vi "Digital chip test.vi"() -> ()   [LabVIEW 2019]
uses:
  <vilib>/Utility/error.llb/DialogType.ctl
  <vilib>/VirtualBench/_DMM Configure Measurement2.vi
  <vilib>/VirtualBench/_PS Configure Voltage Output0.vi
  <vilib>/VirtualBench/_FGEN Configure Standard Waveform4.vi
  <vilib>/VirtualBench/_MSO Configure Analog Channel28.vi
  <vilib>/VirtualBench/_MSO Configure Timing12.vi
  <vilib>/VirtualBench/VirtualBench.lvlib
  <vilib>/DigilentWF/DigilentWF.lvlib
panel:
  out "VOL(V)":dbl=0.31394030101314113 format="%#.2f"
  in  "图表选项卡":enum32{"VOH", "VOL", "电压传输特性"}(tab)=enum."电压传输特性"
  out "VOH":string[][](table)=[["4.750000", "0.100000", "-400.366771", "3.323930"]]
  out "VOL(V)":string[][](table)=[["4.750000", "0.100000", "1.870034", "0.313940"]]
  out "波形图":waveform(dbl)[](graph)=[{"t0"=timestamp(3807570457.144273 s since 1904-01-01), "dt"=1e-06, "Y"=array[5001 elements], "attributes"=variant("NI_ChannelName"=variant(string "mso/1"), "NI_UnitDescription"=variant(string "Volts"))}, {"t0"=timestamp(3807570457.144273 s since 1904-01-01), "dt"=1e-06, "Y"=array[5001 elements], "attributes"=variant("NI_ChannelName"=variant(string "mso/2"), "NI_UnitDescription"=variant(string "Volts"))}]
  out "VOH(V)":dbl=3.3239303310872046 format="%#.2f"
  out "IIH(μA)":dbl=1.1257554185044154 format="%#.2f"
  out "IIL(mA)":dbl=-0.1878597460447979 format="%#.2f"
  out "ICCH(mA)":dbl=0.8908473136992855 format="%#.2f"
  in  "测试参数选项卡":T1(tab)=enum."VOL"
  in  "通道一电压":T2={"+6V通道"="ADP5250-32C0AAE/ps/+6V", "Voltage Level"=5.25, "Current Limit"=0.1}
  in  "测量模式":T3(ring)=enum."DC Current"
  in  "通道一电压 2":T2={"+6V通道"="ADP5250-32C0AAE/ps/+6V", "Voltage Level"=5.25, "Current Limit"=0.1}
  in  "测量模式":T3(ring)=enum."DC Current"
  in  "通道一电压":T2={"+6V通道"="ADP5250-32C0AAE/ps/+6V", "Voltage Level"=5.25, "Current Limit"=0.1}
  in  "测量模式":T3(ring)=enum."DC Current"
  in  "通道一电压 3":T4={"+25V通道"="ADP5250-32C0AAE/ps/+25V", "Voltage Level"=0.4, "Current Limit"=0.1}
  in  "通道一电压":T2={"+6V通道"="ADP5250-32C0AAE/ps/+6V", "Voltage Level"=5.25, "Current Limit"=0.1}
  in  "测量模式":T3(ring)=enum."DC Current"
  in  "通道一电压2":T4={"+25V通道"="ADP5250-32C0AAE/ps/+25V", "Voltage Level"=2.7, "Current Limit"=0.1}
  in  "通道一电压 4":T2={"+6V通道"="ADP5250-32C0AAE/ps/+6V", "Voltage Level"=4.75, "Current Limit"=0.1}
  in  "测量模式 2":T3(ring)=enum."DC Current"
  in  "通道一电压2 2":T4={"+25V通道"="ADP5250-32C0AAE/ps/+25V", "Voltage Level"=0.8, "Current Limit"=0.1}
  in  "测量模式":T3(ring)=enum."DC Current"
  in  "通道一电压2 5":T4={"+25V通道"="ADP5250-32C0AAE/ps/+25V", "Voltage Level"=2.0, "Current Limit"=0.1}
  in  "通道一电压 6":T2={"+6V通道"="ADP5250-32C0AAE/ps/+6V", "Voltage Level"=4.75, "Current Limit"=0.1}
  in  "通道一电压1":T2={"+6V通道"="ADP5250-32C0AAE/ps/+6V", "Voltage Level"=5.0, "Current Limit"=0.1}
  in  "通道一电压2 4":T4={"+25V通道"="ADP5250-32C0AAE/ps/+25V", "Voltage Level"=5.0, "Current Limit"=0.1}
  in  "Amplitude":dbl=4.8 caption="Amplitude (no change)"
  in  "DC Offset":dbl=2.4 caption="DC Offset (no change)"
  in  "测量范围":dbl=5.0 caption="Vertical Range (no change)"
  in  "示波器通道选择":tag="mso/1:2" caption="Channel"
  in  "Waveform Function":i32(ring)=2 caption="Waveform Function (no change)" items=["Sine", "Square", "Triangle/Ramp", "DC"]
  in  "Frequency":dbl=1000.0 caption="Frequency (no change)"
  out "ICCL(mA)":dbl=2.7849634374747283 format="%#.2f"
  in  "测试机台选择":tag="ADP5250-32C0AAE"
  in  "开始测试":bool caption="Start"
  out "测试进度":u8(slide)=100 caption="Testing..." scale=0.0..100.0
  # "基于IECUBE-3839的74芯片自动化测试程序"
  # "硬件配置"
  # "DUT测试参数"
  # "电源配置"
  # "数字万用表配置"
  # "电源配置"
  # "数字万用表配置"
  # "电源配置"
  # "数字万用表配置"
  # "电源配置"
  # "数字万用表配置"
  # "电源配置"
  # "数字万用表配置"
  # "电源配置"
  # "数字万用表配置"
  # "电源配置"
  # "信号源配置"
  # "示波器配置"
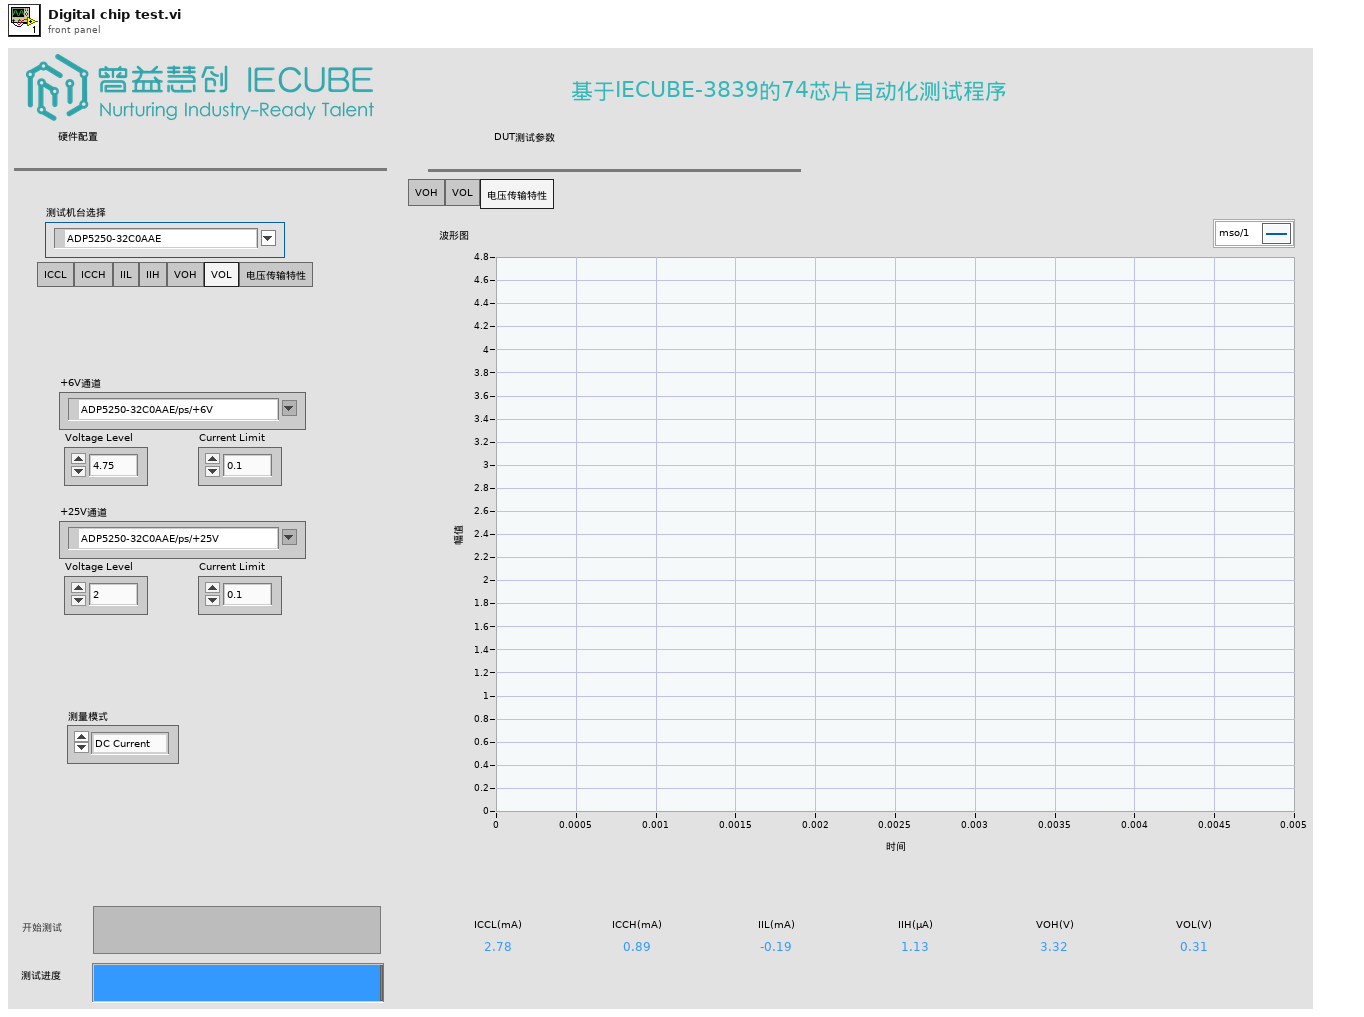
[diagram p1: front panel]
types:
  T1 = enum32{"ICCL", "ICCH", "IIL", "IIH", "VOH", "VOL", "电压传输特性"}
  T2 = cluster{"+6V通道":tag, "Voltage Level":dbl, "Current Limit":dbl}
  T3 = enum16{"DC Volts", "AC Volts", "DC Current", "AC Current", "Resistance", "Diode"}
  T4 = cluster{"+25V通道":tag, "Voltage Level":dbl, "Current Limit":dbl}
  T5 = typedef "枚举.ctl" = enum16{"ICCL", "ICCH", "IIL", "IIH", "VOH", "VOL", "电压传输特性"}
  T6 = typedef "DialogType.ctl" = u16
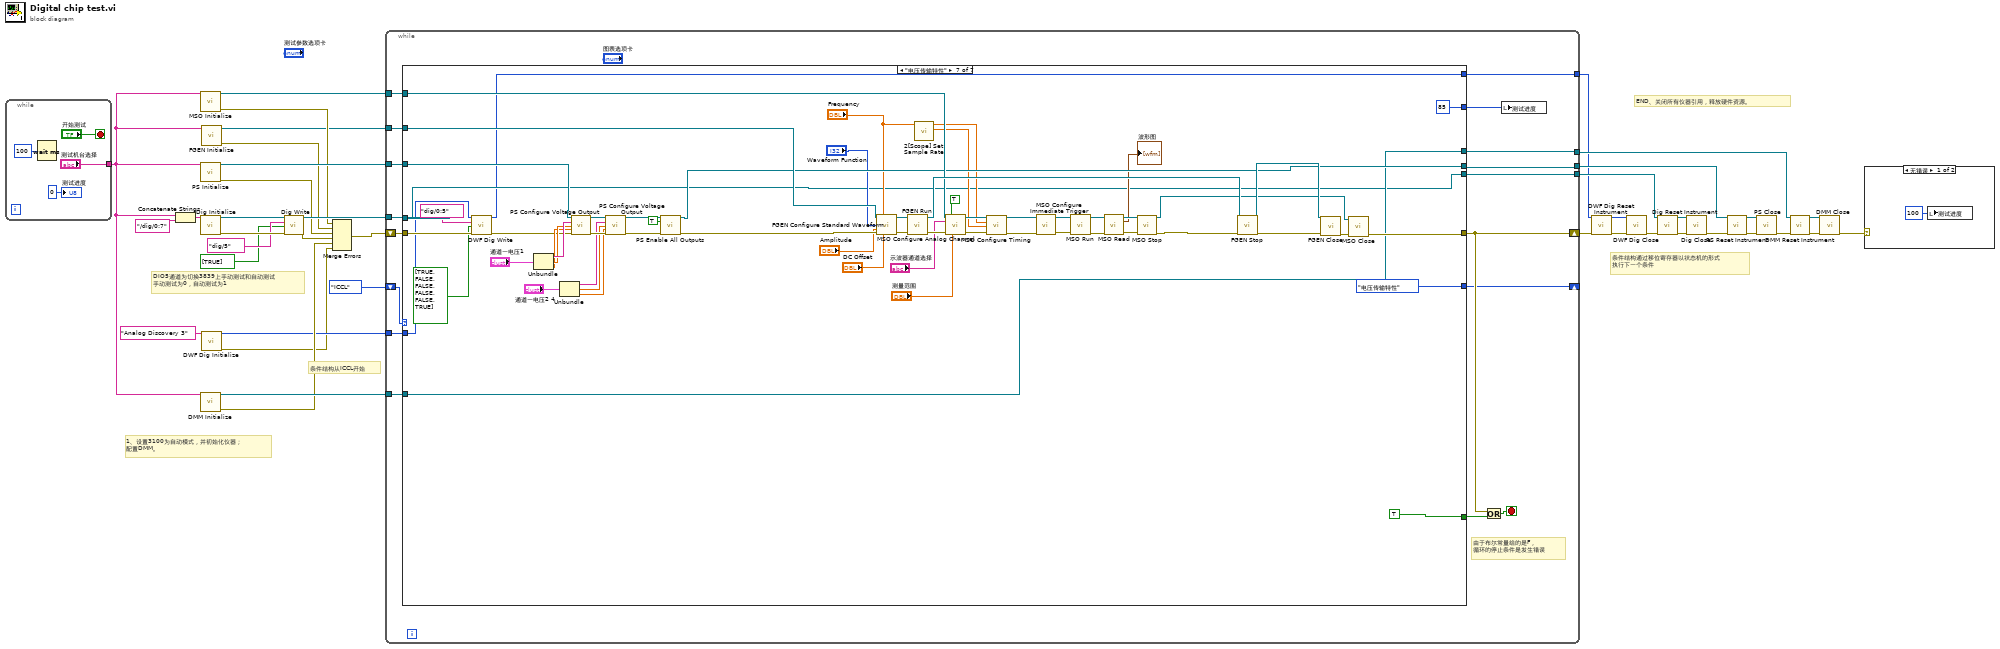
[diagram p0: block diagram]
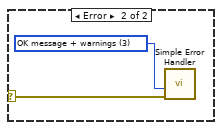
[diagram p2: hidden frame]
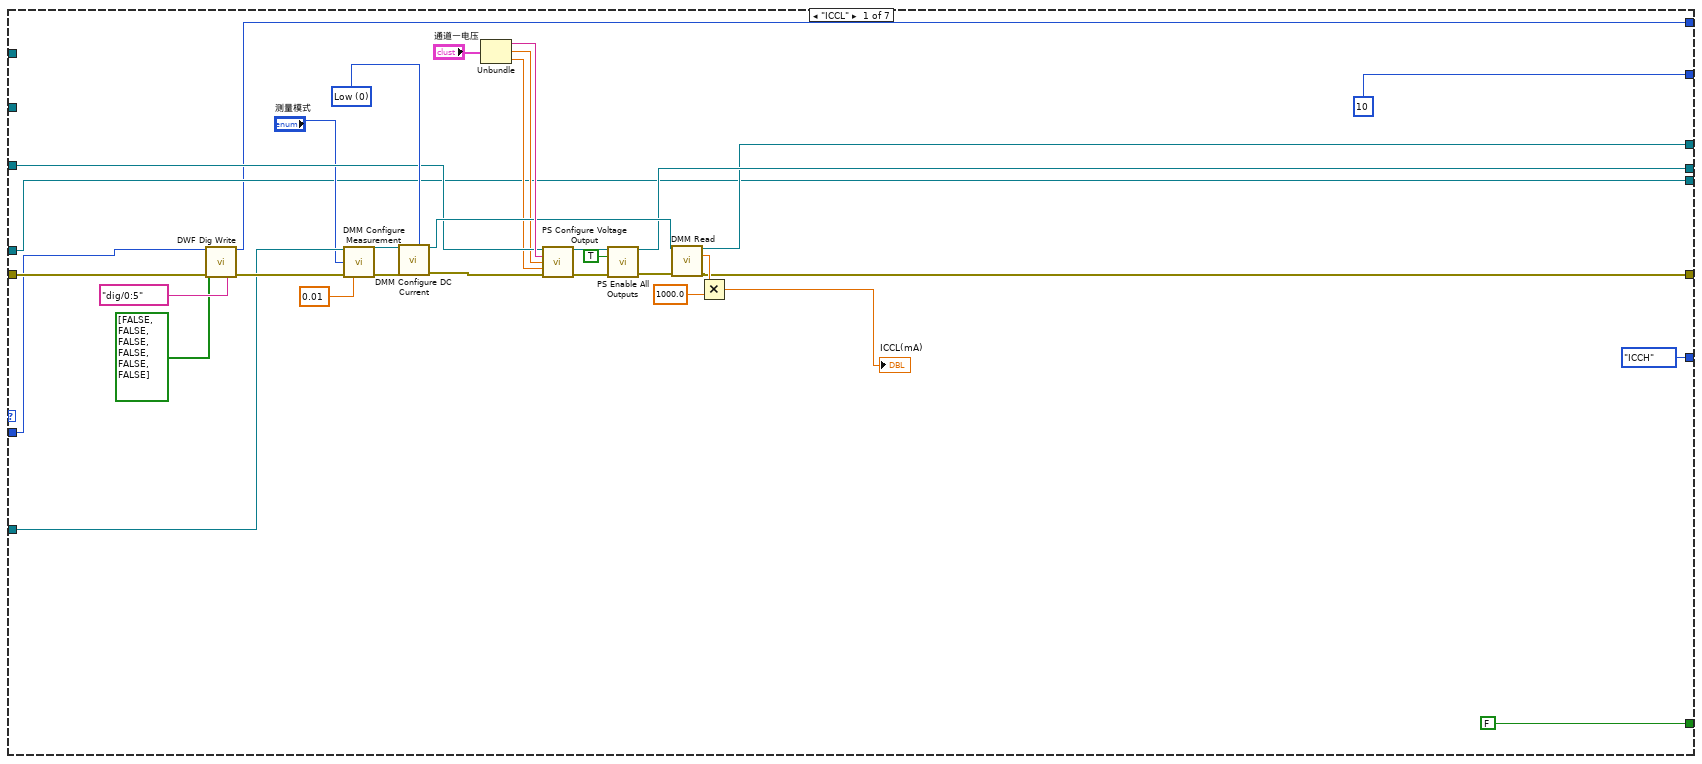
[diagram p3: hidden frame]
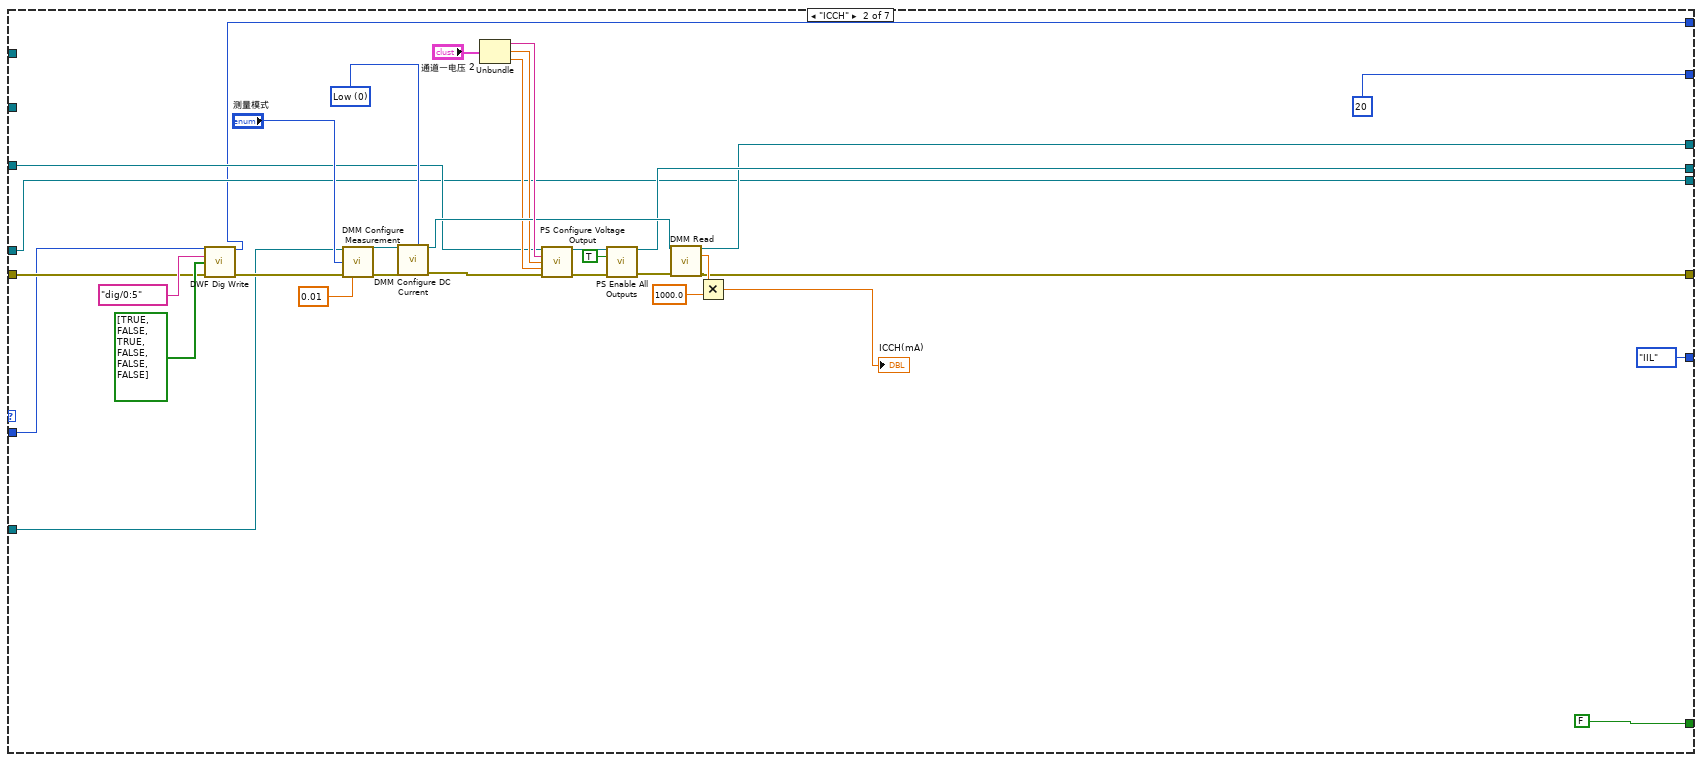
[diagram p4: hidden frame]
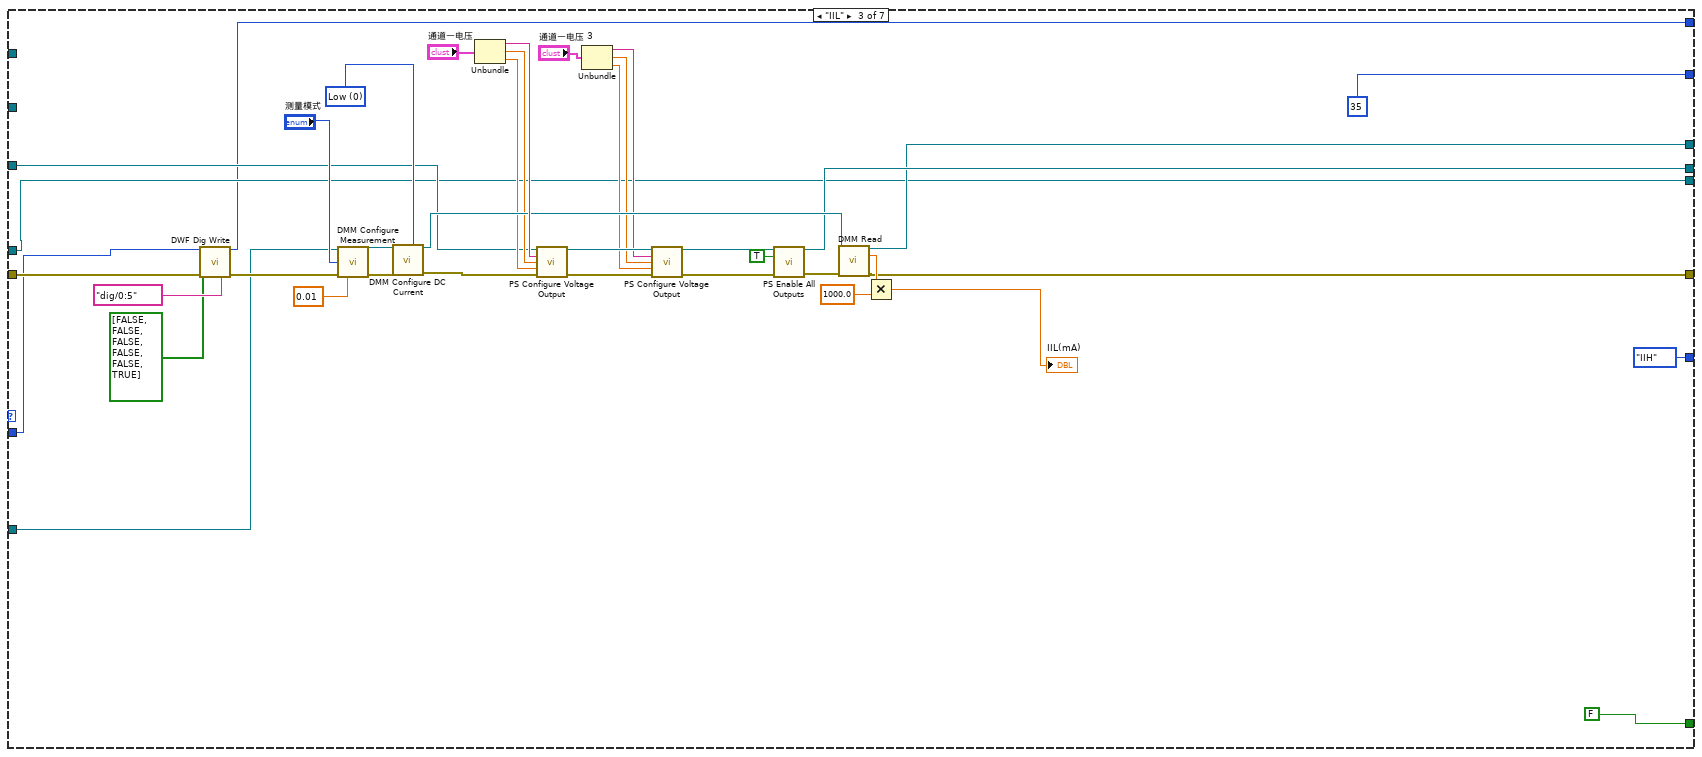
[diagram p5: hidden frame]
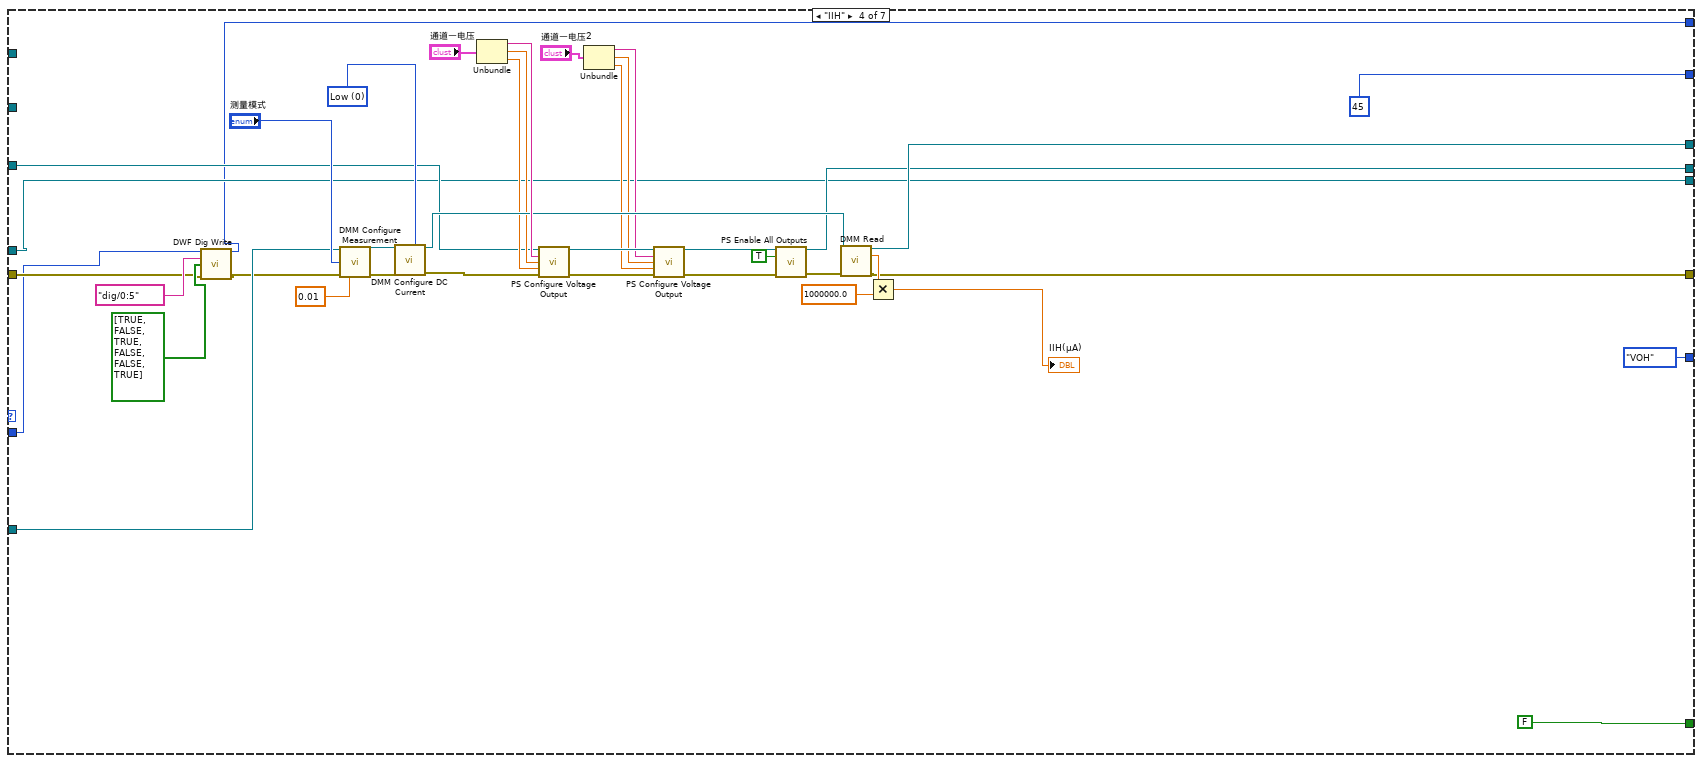
[diagram p6: hidden frame]
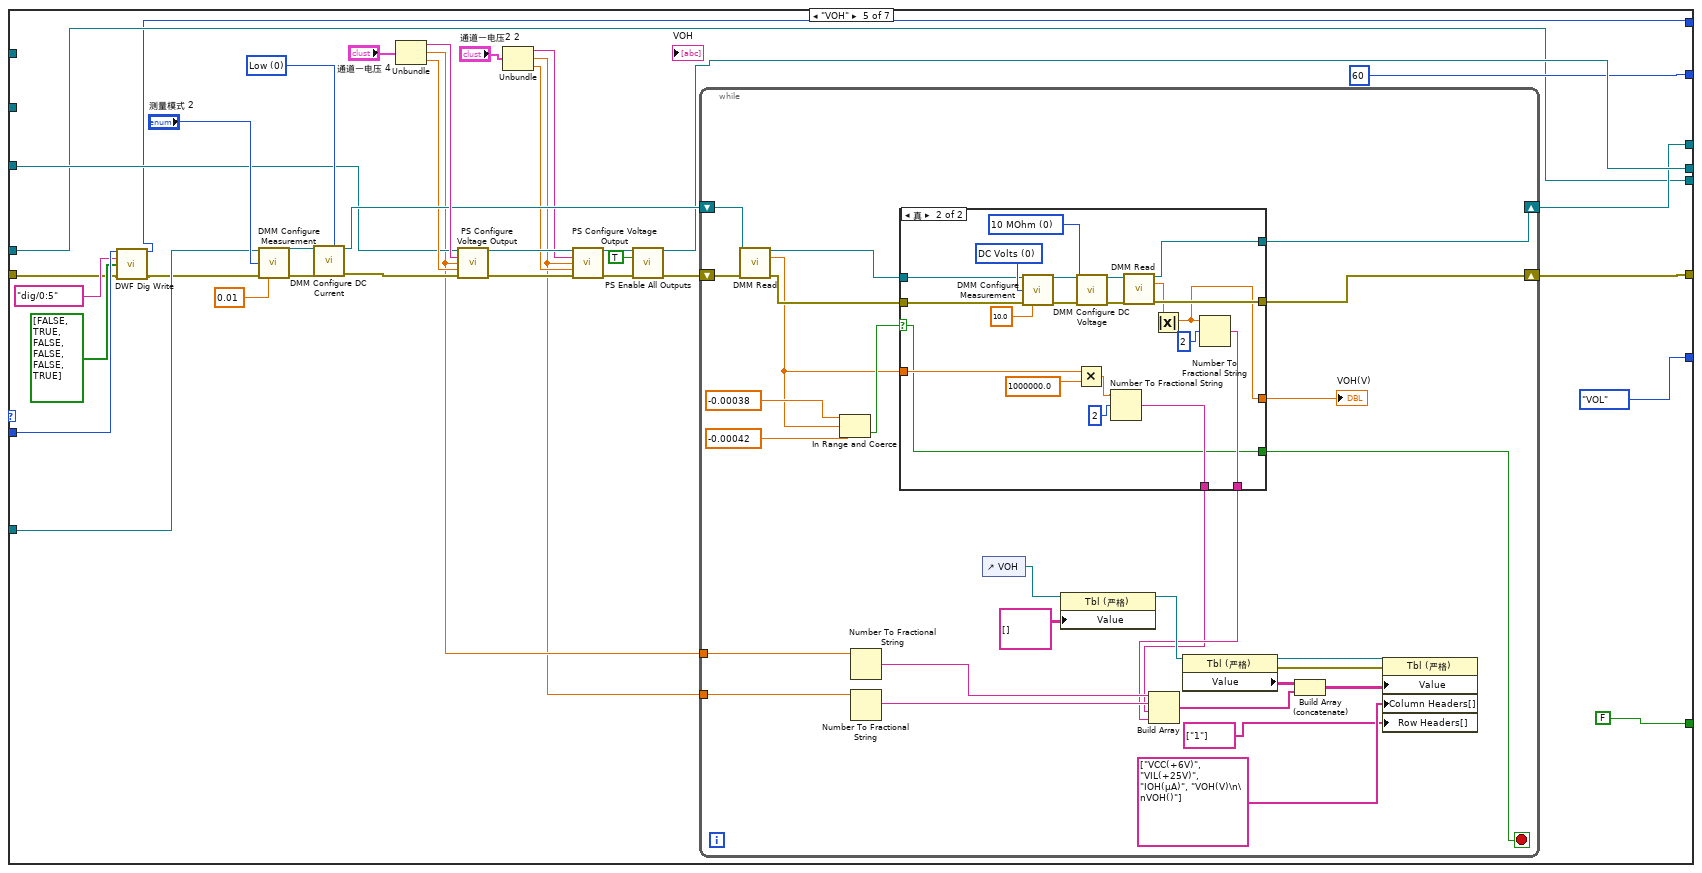
[diagram p7: hidden frame]
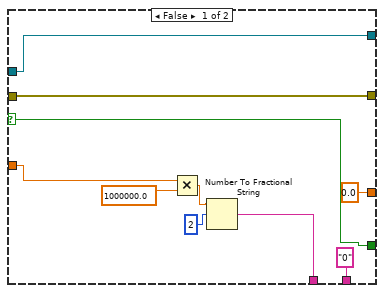
[diagram p8: hidden frame]
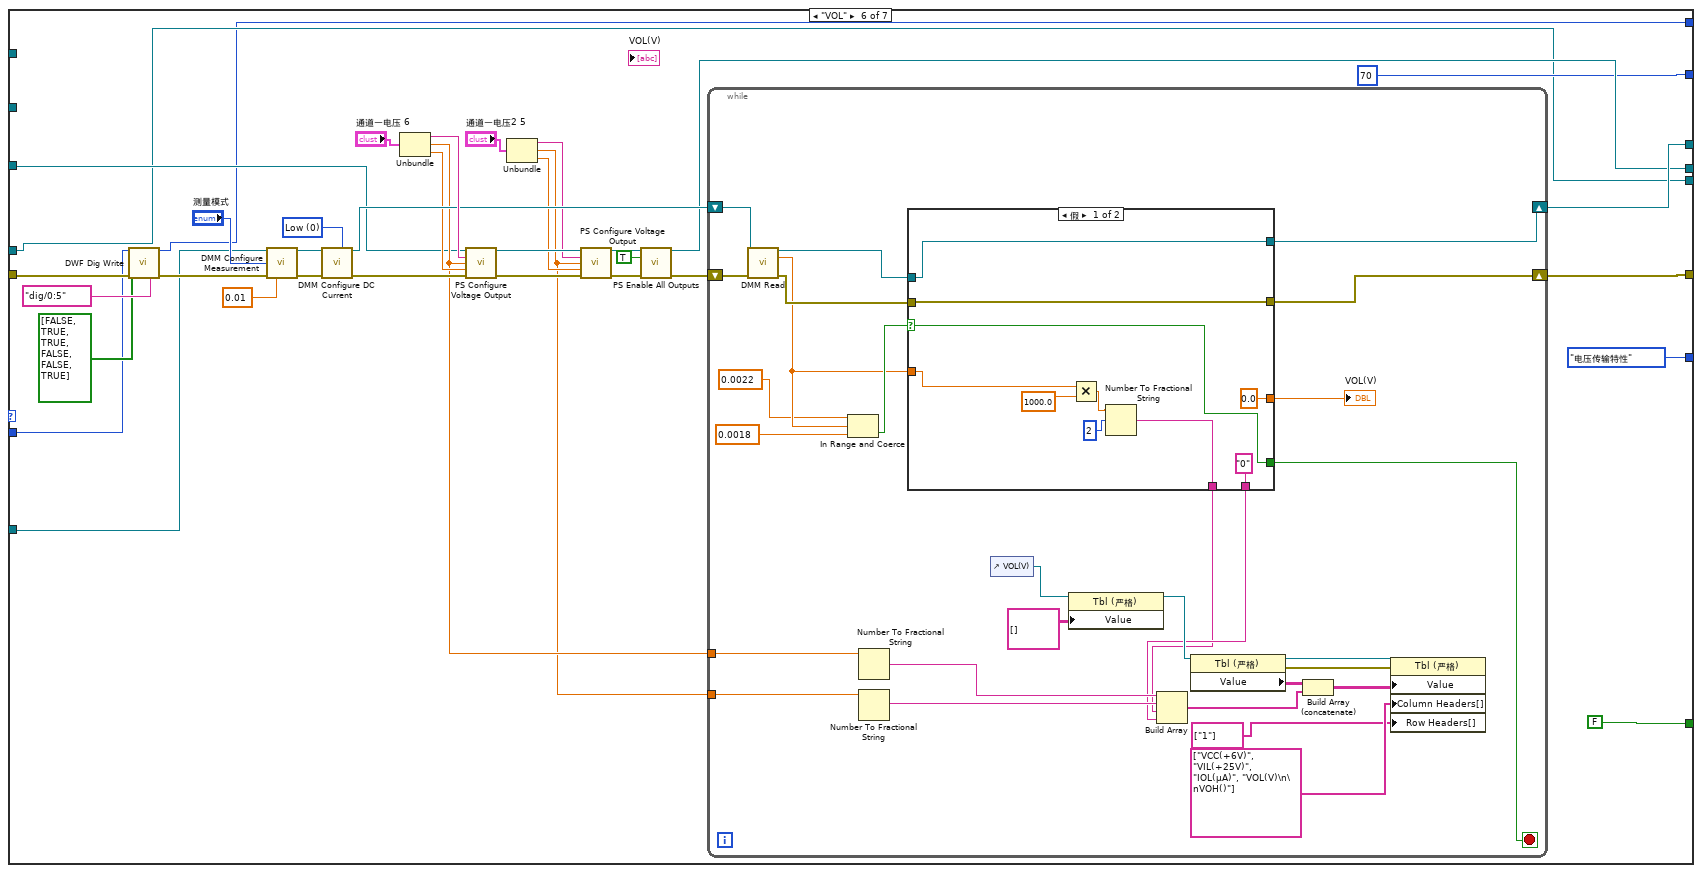
[diagram p9: hidden frame]
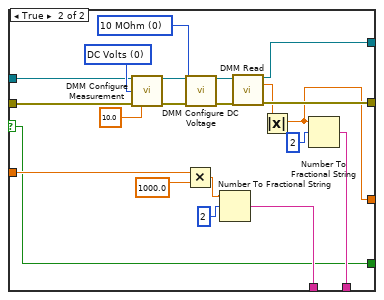
[diagram p10: hidden frame]
diagram:
  # "条件结构通过移位寄存器以状态机的形式\n执行下一个条件"
  # "条件结构从ICCL开始"
  # "DIO5通道为切换3839上手动测试和自动测试\n手动测试为0，自动测试为1"
  # "END、关闭所有仪器引用，释放硬件资源。"
  # "1、设置3100为自动模式，并初始化仪器；\n配置DMM。"
  n1 = while {
    tunnel: ["测试机台选择"] -> w14
    stop <- "开始测试" stop-if-true
    n2 = Wait (ms)(milliseconds to wait=u32 100 ("等待时间（毫秒）")) -> ()  [unwired: 1 out]
    "测试进度" <- u8 0 ("测试进度")
  }
  n3 = Concatenate Strings(w14, "/dig/0:7" ("字符串")) -> (w34:string)
  n4 = call <vilib>:"MSO Initialize.vi"("Device Name"=w14) -> ("Instrument Handle Out"=w11:refnum<k21>, "Error Out"=w12:errorcluster)  [unwired: 13 in]
  n5 = call <vilib>:"PS Initialize.vi"("Device Name"=w14) -> ("Instrument Handle Out"=w33:refnum<k21>, "Error Out"=w30:errorcluster)  [unwired: 13 in]
  n6 = call <vilib>:"Dig Initialize.vi"("Lines"=w34) -> ("Instrument Handle Out"=w39:refnum<k21>, "Error Out"=w38:errorcluster)  [unwired: 13 in]
  n7 = call <vilib>:"DMM Initialize.vi"("Device Name"=w14) -> ("Instrument Handle Out"=w28:refnum<k21>, "Error Out"=w27:errorcluster)  [unwired: 13 in]
  n8 = call <vilib>:"FGEN Initialize.vi"("Device Name"=w14) -> ("Instrument Handle Out"=w10:refnum<k21>, "Error Out"=w13:errorcluster)  [unwired: 13 in]
  n9 = call <vilib>:"DWF Dig Initialize.vi"("Device Name/Lines"="Analog Discovery 3") -> ("Instrument Handle Out"=w7:u32, "Error Out"=w6:errorcluster)  [unwired: 13 in]
  n10 = call <vilib>:"Dig Write.vi"("Instrument Handle In"=w39, "Lines"=tag "dig/5", "Data"=bool[] [TRUE], "Error In"=w38) -> ("Instrument Handle Out"=w32:refnum<k21>, "Error Out"=w29:errorcluster)  [unwired: 10 in]
  n11 = Merge Errors(w12, w13, w30, w29, w27, w6) -> (w31:errorcluster)
  n12 = while {
    tunnel: w32 -> [w58]
    tunnel: w33 -> [w57]
    tunnel: w28 -> [w60]
    shift-right: [w51] -> w5
    shift-left: w31 -> [w59]
    tunnel: [w50] -> w17
    tunnel: [w56] -> w23
    tunnel: [w52] -> w15
    tunnel: w11 -> [w49]
    tunnel: w10 -> [w48]
    shift-right: [w46] -> _
    shift-left: 枚举."ICCL" -> [w47]
    tunnel: w7 -> [w45]
    tunnel: [w44] -> w2
    stop <- w53 stop-if-true
    # "由于布尔常量给的是F，\n循环的停止条件是发生错误"
    n13 = case shown="\"电压传输特性\"" w47 {
      tunnel: w60 -> [w76 w103 w144 w179 w221 w312 w410]
      tunnel: w59 -> [w78 w104 w145 w169 w208 w313 w422]
      tunnel: w58 -> [w63 w96 w129 w172 w212 w303 w397]
      tunnel: w57 -> [w74 w105 w146 w180 w222 w314 w419]
      tunnel: [w65 w101 w141 w177 w218 w310 w410] -> w50
      tunnel: [w73 w102 w142 w176 w219 w309 w413] -> w56
      tunnel: [u8 10 ("测试进度") u8 20 ("测试进度") u8 35 ("测试进度") u8 45 ("测试进度") u8 60 ("测试进度") u8 70 ("测试进度") u8 85 ("测试进度")] -> w55
      tunnel: [FALSE FALSE FALSE FALSE FALSE FALSE TRUE] -> w54
      tunnel: [w63 w96 w129 w172 w212 w303 w397] -> w52
      tunnel: [w66 w99 w143 w175 w220 w311 w411] -> w51
      tunnel: w49 -> [_ _ _ _ _ _ w416]
      tunnel: w48 -> [_ _ _ _ _ _ w415]
      tunnel: [枚举."ICCH" ("枚举") 枚举."IIL" ("枚举") 枚举."IIH" ("枚举") 枚举."VOH" ("枚举") 枚举."VOL" ("枚举") 枚举."电压传输特性" ("枚举") 枚举."电压传输特性" ("枚举")] -> w46
      tunnel: w45 -> [w62 w95 w128 w167 w211 w302 w396]
      tunnel: [w61 w94 w127 w166 w206 w301 w395] -> w44
      frame "ICCL" {
        w90 = 0 items=["Low", "High"] ("Auto Range Terminal")
        n14 = call <vilib>:"DWF Dig Write.vi"("Instrument Handle In"=w62, "Lines"=tag "dig/0:5", "Data"=bool[] [FALSE, FALSE, FALSE, FALSE, FALSE, FALSE], "Error In"=w78) -> ("Instrument Handle Out"=w61:u32, "Error Out"=w77:errorcluster)  [unwired: 10 in]
        n15 = call-poly <vilib>:"DMM Configure Measurement.vi"("Instrument Handle In"=w76, "Function"="测量模式", "Error In"=w77, "Manual Range"=0.01) -> ("Instrument Handle Out"=w91:refnum<k21>, "Error Out"=w92:errorcluster)  [unwired: 10 in]
        n16 = call <vilib>:"DMM Configure DC Current.vi"("Instrument Handle In"=w91, "Auto Range Terminal"=w90, "Error In"=w92) -> ("Instrument Handle Out"=w82:refnum<k21>, "Error Out"=w75:errorcluster)  [unwired: 11 in]
        n17 = Unbundle("通道一电压") -> ("+6V通道"=w86:tag, "Voltage Level"=w68:dbl, "Current Limit"=w69:dbl)
        n18 = call-poly <vilib>:"PS Configure Voltage Output.vi"("Instrument Handle In"=w74, "Channel"=w86, "Voltage Level"=w68, "Current Limit"=w69, "Error In"=w75) -> ("Instrument Handle Out"=w85:refnum<k21>, "Error Out"=w84:errorcluster)  [unwired: 9 in]
        n19 = call <vilib>:"PS Enable All Outputs.vi"("Instrument Handle In"=w85, "Enable Outputs"=TRUE, "Error In"=w84) -> ("Instrument Handle Out"=w73:refnum<k21>, "Error Out"=w81:errorcluster)  [unwired: 11 in]
        n20 = call <vilib>:"DMM Read.vi"("Instrument Handle In"=w82, "Error In"=w81) -> ("Instrument Handle Out"=w65:refnum<k21>, "Measurement"=w80:dbl, "Error Out"=w66:errorcluster)  [unwired: 11 in]
        n21 = Multiply(x=w80, y=1000.0) -> (x*y=→"ICCL(mA)":dbl)
      }
      frame "ICCH" {
        w124 = 0 items=["Low", "High"] ("Auto Range Terminal")
        n22 = call <vilib>:"DWF Dig Write.vi"("Instrument Handle In"=w95, "Lines"=tag "dig/0:5", "Data"=bool[] [TRUE, FALSE, TRUE, FALSE, FALSE, FALSE], "Error In"=w104) -> ("Instrument Handle Out"=w94:u32, "Error Out"=w112:errorcluster)  [unwired: 10 in]
        n23 = call-poly <vilib>:"DMM Configure Measurement.vi"("Instrument Handle In"=w103, "Function"="测量模式", "Error In"=w112, "Manual Range"=0.01) -> ("Instrument Handle Out"=w125:refnum<k21>, "Error Out"=w126:errorcluster)  [unwired: 10 in]
        n24 = call <vilib>:"DMM Configure DC Current.vi"("Instrument Handle In"=w125, "Auto Range Terminal"=w124, "Error In"=w126) -> ("Instrument Handle Out"=w116:refnum<k21>, "Error Out"=w111:errorcluster)  [unwired: 11 in]
        n25 = Unbundle("通道一电压 2") -> ("+6V通道"=w120:tag, "Voltage Level"=w107:dbl, "Current Limit"=w108:dbl)
        n26 = call-poly <vilib>:"PS Configure Voltage Output.vi"("Instrument Handle In"=w105, "Channel"=w120, "Voltage Level"=w107, "Current Limit"=w108, "Error In"=w111) -> ("Instrument Handle Out"=w119:refnum<k21>, "Error Out"=w118:errorcluster)  [unwired: 9 in]
        n27 = call <vilib>:"PS Enable All Outputs.vi"("Instrument Handle In"=w119, "Enable Outputs"=TRUE, "Error In"=w118) -> ("Instrument Handle Out"=w102:refnum<k21>, "Error Out"=w115:errorcluster)  [unwired: 11 in]
        n28 = call <vilib>:"DMM Read.vi"("Instrument Handle In"=w116, "Error In"=w115) -> ("Instrument Handle Out"=w101:refnum<k21>, "Measurement"=w114:dbl, "Error Out"=w99:errorcluster)  [unwired: 11 in]
        n29 = Multiply(x=w114, y=1000.0) -> (x*y=→"ICCH(mA)":dbl)
      }
      frame "IIL" {
        w163 = 0 items=["Low", "High"] ("Auto Range Terminal")
        n30 = call <vilib>:"DWF Dig Write.vi"("Instrument Handle In"=w128, "Lines"=tag "dig/0:5", "Data"=bool[] [FALSE, FALSE, FALSE, FALSE, FALSE, TRUE], "Error In"=w145) -> ("Instrument Handle Out"=w127:u32, "Error Out"=w153:errorcluster)  [unwired: 10 in]
        n31 = call-poly <vilib>:"DMM Configure Measurement.vi"("Instrument Handle In"=w144, "Function"="测量模式", "Error In"=w153, "Manual Range"=0.01) -> ("Instrument Handle Out"=w164:refnum<k21>, "Error Out"=w165:errorcluster)  [unwired: 10 in]
        n32 = call <vilib>:"DMM Configure DC Current.vi"("Instrument Handle In"=w164, "Auto Range Terminal"=w163, "Error In"=w165) -> ("Instrument Handle Out"=w157:refnum<k21>, "Error Out"=w152:errorcluster)  [unwired: 11 in]
        n33 = Unbundle("通道一电压") -> ("+6V通道"=w159:tag, "Voltage Level"=w148:dbl, "Current Limit"=w149:dbl)
        n34 = call-poly <vilib>:"PS Configure Voltage Output.vi"("Instrument Handle In"=w146, "Channel"=w159, "Voltage Level"=w148, "Current Limit"=w149, "Error In"=w152) -> ("Instrument Handle Out"=w138:refnum<k21>, "Error Out"=w135:errorcluster)  [unwired: 9 in]
        n35 = Unbundle("通道一电压 3") -> ("+25V通道"=w134:tag, "Voltage Level"=w133:dbl, "Current Limit"=w132:dbl)
        n36 = call-poly <vilib>:"PS Configure Voltage Output.vi"("Instrument Handle In"=w138, "Channel"=w134, "Voltage Level"=w133, "Current Limit"=w132, "Error In"=w135) -> ("Instrument Handle Out"=w137:refnum<k21>, "Error Out"=w136:errorcluster)  [unwired: 9 in]
        n37 = call <vilib>:"PS Enable All Outputs.vi"("Instrument Handle In"=w137, "Enable Outputs"=TRUE, "Error In"=w136) -> ("Instrument Handle Out"=w142:refnum<k21>, "Error Out"=w156:errorcluster)  [unwired: 11 in]
        n38 = call <vilib>:"DMM Read.vi"("Instrument Handle In"=w157, "Error In"=w156) -> ("Instrument Handle Out"=w141:refnum<k21>, "Measurement"=w155:dbl, "Error Out"=w143:errorcluster)  [unwired: 11 in]
        n39 = Multiply(x=w155, y=1000.0) -> (x*y=→"IIL(mA)":dbl)
      }
      frame "IIH" {
        w202 = 0 items=["Low", "High"] ("Auto Range Terminal")
        n40 = call <vilib>:"DWF Dig Write.vi"("Instrument Handle In"=w167, "Lines"=tag "dig/0:5", "Data"=bool[] [TRUE, FALSE, TRUE, FALSE, FALSE, TRUE], "Error In"=w169) -> ("Instrument Handle Out"=w166:u32, "Error Out"=w168:errorcluster)  [unwired: 10 in]
        n41 = call-poly <vilib>:"DMM Configure Measurement.vi"("Instrument Handle In"=w179, "Function"="测量模式", "Error In"=w168, "Manual Range"=0.01) -> ("Instrument Handle Out"=w203:refnum<k21>, "Error Out"=w204:errorcluster)  [unwired: 10 in]
        n42 = call <vilib>:"DMM Configure DC Current.vi"("Instrument Handle In"=w203, "Auto Range Terminal"=w202, "Error In"=w204) -> ("Instrument Handle Out"=w198:refnum<k21>, "Error Out"=w194:errorcluster)  [unwired: 11 in]
        n43 = Unbundle("通道一电压") -> ("+6V通道"=w200:tag, "Voltage Level"=w190:dbl, "Current Limit"=w191:dbl)
        n44 = call-poly <vilib>:"PS Configure Voltage Output.vi"("Instrument Handle In"=w180, "Channel"=w200, "Voltage Level"=w190, "Current Limit"=w191, "Error In"=w194) -> ("Instrument Handle Out"=w187:refnum<k21>, "Error Out"=w184:errorcluster)  [unwired: 9 in]
        n45 = Unbundle("通道一电压2") -> ("+25V通道"=w183:tag, "Voltage Level"=w182:dbl, "Current Limit"=w181:dbl)
        n46 = call-poly <vilib>:"PS Configure Voltage Output.vi"("Instrument Handle In"=w187, "Channel"=w183, "Voltage Level"=w182, "Current Limit"=w181, "Error In"=w184) -> ("Instrument Handle Out"=w186:refnum<k21>, "Error Out"=w185:errorcluster)  [unwired: 9 in]
        n47 = call <vilib>:"PS Enable All Outputs.vi"("Instrument Handle In"=w186, "Enable Outputs"=TRUE, "Error In"=w185) -> ("Instrument Handle Out"=w176:refnum<k21>, "Error Out"=w197:errorcluster)  [unwired: 11 in]
        n48 = call <vilib>:"DMM Read.vi"("Instrument Handle In"=w198, "Error In"=w197) -> ("Instrument Handle Out"=w177:refnum<k21>, "Measurement"=w196:dbl, "Error Out"=w175:errorcluster)  [unwired: 11 in]
        n49 = Multiply(x=w196, y=1000000.0) -> (x*y=→"IIH(μA)":dbl)
      }
      frame "VOH" {
        w238 = 0 items=["Low", "High"] ("Auto Range Terminal")
        n50 = call <vilib>:"DWF Dig Write.vi"("Instrument Handle In"=w211, "Lines"=tag "dig/0:5", "Data"=bool[] [FALSE, TRUE, FALSE, FALSE, FALSE, TRUE], "Error In"=w208) -> ("Instrument Handle Out"=w206:u32, "Error Out"=w207:errorcluster)  [unwired: 10 in]
        n51 = call-poly <vilib>:"DMM Configure Measurement.vi"("Instrument Handle In"=w221, "Function"="测量模式 2", "Error In"=w207, "Manual Range"=0.01) -> ("Instrument Handle Out"=w239:refnum<k21>, "Error Out"=w240:errorcluster)  [unwired: 10 in]
        n52 = call <vilib>:"DMM Configure DC Current.vi"("Instrument Handle In"=w239, "Auto Range Terminal"=w238, "Error In"=w240) -> ("Instrument Handle Out"=w234:refnum<k21>, "Error Out"=w232:errorcluster)  [unwired: 11 in]
        n53 = Unbundle("通道一电压 4") -> ("+6V通道"=w236:tag, "Voltage Level"=w216:dbl, "Current Limit"=w230:dbl)
        n54 = call-poly <vilib>:"PS Configure Voltage Output.vi"("Instrument Handle In"=w222, "Channel"=w236, "Voltage Level"=w216, "Current Limit"=w230, "Error In"=w232) -> ("Instrument Handle Out"=w227:refnum<k21>, "Error Out"=w224:errorcluster)  [unwired: 9 in]
        n55 = Unbundle("通道一电压2 2") -> ("+25V通道"=w223:tag, "Voltage Level"=w205:dbl, "Current Limit"=w215:dbl)
        n56 = call-poly <vilib>:"PS Configure Voltage Output.vi"("Instrument Handle In"=w227, "Channel"=w223, "Voltage Level"=w205, "Current Limit"=w215, "Error In"=w224) -> ("Instrument Handle Out"=w226:refnum<k21>, "Error Out"=w225:errorcluster)  [unwired: 9 in]
        n57 = call <vilib>:"PS Enable All Outputs.vi"("Instrument Handle In"=w226, "Enable Outputs"=TRUE, "Error In"=w225) -> ("Instrument Handle Out"=w219:refnum<k21>, "Error Out"=w233:errorcluster)  [unwired: 11 in]
        n58 = while {
          shift-right: [w261] -> w218
          shift-left: w234 -> [w268]
          shift-right: [w260] -> w220
          shift-left: w233 -> [w267]
          tunnel: w216 -> [w244]
          tunnel: w205 -> [w243]
          stop <- w241 stop-if-true
          n59 = call <vilib>:"DMM Read.vi"("Instrument Handle In"=w268, "Error In"=w267) -> ("Instrument Handle Out"=w263:refnum<k21>, "Measurement"=w259:dbl, "Error Out"=w262:errorcluster)  [unwired: 11 in]
          n60 = In Range and Coerce(upper limit=-0.00038 ("上限"), x=w259, lower limit=-0.00042 ("下限")) -> (In Range?=w264:bool)  [unwired: 1 out]
          n61 = Number To Fractional String(number=w244) -> (F-format string=w258:string)  [unwired: 3 in]
          n62 = Number To Fractional String(number=w243) -> (F-format string=w251:string)  [unwired: 3 in]
          n63 = case shown="真" w264 {
            selector: w264 -> [w269 w280]
            tunnel: w263 -> [w278 w288]
            tunnel: w262 -> [w277 w287]
            tunnel: [w278 w286] -> w261
            tunnel: [w277 w285] -> w260
            tunnel: w259 -> [w274 w284]
            tunnel: ["0" w283] -> w246
            tunnel: [w273 w282] -> w245
            tunnel: [0.0 ("Measurement") w279] -> w242
            tunnel: [w269 w280] -> w241
            frame False {
              n64 = Multiply(x=w274, y=1000000.0) -> (x*y=w271:dbl)
              n65 = Number To Fractional String(number=w271, width (-)=i16 2 ("精度(6)")) -> (F-format string=w273:string)  [unwired: 2 in]
            }
            frame True {
              w289 = 0 items=["10 MOhm", "10 GOhm"] ("Input Resistance")
              w296 = 0 items=["DC Volts", "AC Volts", "DC Current", "AC Current", "Resistance", "Diode"] ("Function")
              n66 = call-poly <vilib>:"DMM Configure Measurement.vi"("Instrument Handle In"=w288, "Function"=w296, "Error In"=w287, "Manual Range"=10.0) -> ("Instrument Handle Out"=w294:refnum<k21>, "Error Out"=w293:errorcluster)  [unwired: 10 in]
              n67 = Multiply(x=w284, y=1000000.0) -> (x*y=w299:dbl)
              n68 = call <vilib>:"DMM Configure DC Voltage.vi"("Instrument Handle In"=w294, "Input Resistance"=w289, "Error In"=w293) -> ("Instrument Handle Out"=w292:refnum<k21>, "Error Out"=w291:errorcluster)  [unwired: 11 in]
              n69 = Number To Fractional String(number=w299, width (-)=i16 2 ("精度(6)")) -> (F-format string=w282:string)  [unwired: 2 in]
              n70 = call <vilib>:"DMM Read.vi"("Instrument Handle In"=w292, "Error In"=w291) -> ("Instrument Handle Out"=w286:refnum<k21>, "Measurement"=w281:dbl, "Error Out"=w285:errorcluster)  [unwired: 11 in]
              n71 = Absolute Value(x=w281) -> (abs(x)=w279:dbl)
              n72 = Number To Fractional String(number=w279, width (-)=i16 2 ("精度(6)")) -> (F-format string=w283:string)  [unwired: 2 in]
            }
          }
          "VOH(V)" <- w242
          n73 = control-ref of="VOH"() -> (w247:refnum<vi>)
          n74 = property class="Tbl (严格)"(reference=w247, "Value"=string[][] [] ("值")) -> (reference out=w253:refnum<vi>)  [unwired: 1 in, 1 out]
          n75 = Build Array(w258, w251, w245, w246) -> (w252:string[])
          n76 = property class="Tbl (严格)"(reference=w253) -> (reference out=w256:refnum<vi>, error out=w257:errorcluster, "Value"=w255:string[][])  [unwired: 1 in]
          n77 = Build Array (concatenate)(w255, w252) -> (w254:string[][])
          n78 = property class="Tbl (严格)"(reference=w256, error in=w257, "Value"=w254, "Column Headers[]"=string[] ["VCC(+6V)", "VIL(+25V)", "IOH(μA)", "VOH(V)\n\nVOH()"] ("列首字符串[]"), "Row Headers[]"=string[] ["1"] ("列首字符串[]")) -> ()  [unwired: 2 out]
        }
      }
      frame "VOL" {
        w333 = 0 items=["Low", "High"] ("Auto Range Terminal")
        n79 = call <vilib>:"DWF Dig Write.vi"("Instrument Handle In"=w302, "Lines"=tag "dig/0:5", "Data"=bool[] [FALSE, TRUE, TRUE, FALSE, FALSE, TRUE], "Error In"=w313) -> ("Instrument Handle Out"=w301:u32, "Error Out"=w325:errorcluster)  [unwired: 10 in]
        n80 = call-poly <vilib>:"DMM Configure Measurement.vi"("Instrument Handle In"=w312, "Function"="测量模式", "Error In"=w325, "Manual Range"=0.01) -> ("Instrument Handle Out"=w334:refnum<k21>, "Error Out"=w335:errorcluster)  [unwired: 10 in]
        n81 = call <vilib>:"DMM Configure DC Current.vi"("Instrument Handle In"=w334, "Auto Range Terminal"=w333, "Error In"=w335) -> ("Instrument Handle Out"=w327:refnum<k21>, "Error Out"=w324:errorcluster)  [unwired: 11 in]
        n82 = Unbundle("通道一电压 6") -> ("+6V通道"=w329:tag, "Voltage Level"=w316:dbl, "Current Limit"=w322:dbl)
        n83 = call-poly <vilib>:"PS Configure Voltage Output.vi"("Instrument Handle In"=w314, "Channel"=w329, "Voltage Level"=w316, "Current Limit"=w322, "Error In"=w324) -> ("Instrument Handle Out"=w321:refnum<k21>, "Error Out"=w318:errorcluster)  [unwired: 9 in]
        n84 = Unbundle("通道一电压2 5") -> ("+25V通道"=w317:tag, "Voltage Level"=w300:dbl, "Current Limit"=w315:dbl)
        n85 = call-poly <vilib>:"PS Configure Voltage Output.vi"("Instrument Handle In"=w321, "Channel"=w317, "Voltage Level"=w300, "Current Limit"=w315, "Error In"=w318) -> ("Instrument Handle Out"=w320:refnum<k21>, "Error Out"=w319:errorcluster)  [unwired: 9 in]
        n86 = call <vilib>:"PS Enable All Outputs.vi"("Instrument Handle In"=w320, "Enable Outputs"=TRUE, "Error In"=w319) -> ("Instrument Handle Out"=w309:refnum<k21>, "Error Out"=w326:errorcluster)  [unwired: 11 in]
        n87 = while {
          shift-right: [w358] -> w310
          shift-left: w327 -> [w363]
          shift-right: [w357] -> w311
          shift-left: w326 -> [w362]
          tunnel: w316 -> [w341]
          tunnel: w300 -> [w340]
          stop <- w338 stop-if-true
          n88 = call <vilib>:"DMM Read.vi"("Instrument Handle In"=w363, "Error In"=w362) -> ("Instrument Handle Out"=w360:refnum<k21>, "Measurement"=w356:dbl, "Error Out"=w359:errorcluster)  [unwired: 11 in]
          n89 = In Range and Coerce(upper limit=0.0022 ("下限"), x=w356, lower limit=0.0018 ("上限")) -> (In Range?=w361:bool)  [unwired: 1 out]
          n90 = Number To Fractional String(number=w341) -> (F-format string=w355:string)  [unwired: 3 in]
          n91 = Number To Fractional String(number=w340) -> (F-format string=w348:string)  [unwired: 3 in]
          n92 = case shown="假" w361 {
            selector: w361 -> [w364 w375]
            tunnel: w360 -> [w373 w383]
            tunnel: w359 -> [w372 w382]
            tunnel: [w373 w381] -> w358
            tunnel: [w372 w380] -> w357
            tunnel: w356 -> [w369 w379]
            tunnel: ["0" w378] -> w343
            tunnel: [w368 w377] -> w342
            tunnel: [0.0 ("Measurement") w374] -> w339
            tunnel: [w364 w375] -> w338
            frame False {
              n93 = Multiply(x=w369, y=1000.0) -> (x*y=w366:dbl)
              n94 = Number To Fractional String(number=w366, width (-)=i16 2 ("精度(6)")) -> (F-format string=w368:string)  [unwired: 2 in]
            }
            frame True {
              w384 = 0 items=["10 MOhm", "10 GOhm"] ("Input Resistance")
              w391 = 0 items=["DC Volts", "AC Volts", "DC Current", "AC Current", "Resistance", "Diode"] ("Function")
              n95 = call-poly <vilib>:"DMM Configure Measurement.vi"("Instrument Handle In"=w383, "Function"=w391, "Error In"=w382, "Manual Range"=10.0) -> ("Instrument Handle Out"=w389:refnum<k21>, "Error Out"=w388:errorcluster)  [unwired: 10 in]
              n96 = Multiply(x=w379, y=1000.0) -> (x*y=w394:dbl)
              n97 = call <vilib>:"DMM Configure DC Voltage.vi"("Instrument Handle In"=w389, "Input Resistance"=w384, "Error In"=w388) -> ("Instrument Handle Out"=w387:refnum<k21>, "Error Out"=w386:errorcluster)  [unwired: 11 in]
              n98 = Number To Fractional String(number=w394, width (-)=i16 2 ("精度(6)")) -> (F-format string=w377:string)  [unwired: 2 in]
              n99 = call <vilib>:"DMM Read.vi"("Instrument Handle In"=w387, "Error In"=w386) -> ("Instrument Handle Out"=w381:refnum<k21>, "Measurement"=w376:dbl, "Error Out"=w380:errorcluster)  [unwired: 11 in]
              n100 = Absolute Value(x=w376) -> (abs(x)=w374:dbl)
              n101 = Number To Fractional String(number=w374, width (-)=i16 2 ("精度(6)")) -> (F-format string=w378:string)  [unwired: 2 in]
            }
          }
          "VOL(V)" <- w339
          n102 = control-ref of="VOL(V)"() -> (w344:refnum<vi>)
          n103 = property class="Tbl (严格)"(reference=w344, "Value"=string[][] [] ("值")) -> (reference out=w350:refnum<vi>)  [unwired: 1 in, 1 out]
          n104 = Build Array(w355, w348, w342, w343) -> (w349:string[])
          n105 = property class="Tbl (严格)"(reference=w350) -> (reference out=w353:refnum<vi>, error out=w354:errorcluster, "Value"=w352:string[][])  [unwired: 1 in]
          n106 = Build Array (concatenate)(w352, w349) -> (w351:string[][])
          n107 = property class="Tbl (严格)"(reference=w353, error in=w354, "Value"=w351, "Column Headers[]"=string[] ["VCC(+6V)", "VIL(+25V)", "IOL(μA)", "VOL(V)\n\nVOH()"] ("列首字符串[]"), "Row Headers[]"=string[] ["1"] ("列首字符串[]")) -> ()  [unwired: 2 out]
        }
      }
      frame "电压传输特性" {
        n108 = call <vilib>:"DWF Dig Write.vi"("Instrument Handle In"=w396, "Lines"=tag "dig/0:5", "Data"=bool[] [TRUE, FALSE, FALSE, FALSE, FALSE, TRUE], "Error In"=w422) -> ("Instrument Handle Out"=w395:u32, "Error Out"=w414:errorcluster)  [unwired: 10 in]
        n109 = Unbundle("通道一电压1") -> ("+6V通道"=w451:tag, "Voltage Level"=w450:dbl, "Current Limit"=w449:dbl)
        n110 = Unbundle("通道一电压2 4") -> ("+25V通道"=w427:tag, "Voltage Level"=w426:dbl, "Current Limit"=w425:dbl)
        n111 = call-poly <vilib>:"PS Configure Voltage Output.vi"("Instrument Handle In"=w419, "Channel"=w451, "Voltage Level"=w450, "Current Limit"=w449, "Error In"=w414) -> ("Instrument Handle Out"=w445:refnum<k21>, "Error Out"=w446:errorcluster)  [unwired: 9 in]
        n112 = call-poly <vilib>:"PS Configure Voltage Output.vi"("Instrument Handle In"=w445, "Channel"=w427, "Voltage Level"=w426, "Current Limit"=w425) -> ("Instrument Handle Out"=w428:refnum<k21>)  [unwired: 10 in, 1 out]
        n113 = call <vilib>:"PS Enable All Outputs.vi"("Instrument Handle In"=w428, "Enable Outputs"=TRUE, "Error In"=w446) -> ("Instrument Handle Out"=w413:refnum<k21>, "Error Out"=w424:errorcluster)  [unwired: 11 in]
        n114 = call-poly <vilib>:"FGEN Configure Standard Waveform.vi"("Instrument Handle In"=w415, "Frequency"="Frequency", "Waveform Function"="Waveform Function", "Amplitude"="Amplitude", "Error In"=w424, "DC Offset"="DC Offset") -> ("Instrument Handle Out"=w448:refnum<k21>, "Error Out"=w447:errorcluster)  [unwired: 8 in]
        n115 = call <vilib>:"FGEN Run.vi"("Instrument Handle In"=w448, "Error In"=w447) -> ("Instrument Handle Out"=w433:refnum<k21>, "Error Out"=w444:errorcluster)  [unwired: 12 in]
        n116 = call "2[Scope] Set Sample Rate.vi"("Frequency"="Frequency") -> ("Acquistion Time"=w399:dbl, "Sample Rate"=w400:dbl)  [unwired: 9 in]
        n117 = call-poly <vilib>:"MSO Configure Analog Channel.vi"("Instrument Handle In"=w416, "Enable Channel"=TRUE, "Channel"="示波器通道选择", "Error In"=w444, "Vertical Range"="测量范围") -> ("Instrument Handle Out"=w442:refnum<k21>, "Error Out"=w443:errorcluster)  [unwired: 9 in]
        n118 = call-poly <vilib>:"MSO Configure Timing.vi"("Instrument Handle In"=w442, "Sample Rate"=w400, "Acquisition Time (s)"=w399, "Error In"=w443) -> ("Instrument Handle Out"=w441:refnum<k21>, "Error Out"=w440:errorcluster)  [unwired: 10 in]
        n119 = call <vilib>:"MSO Configure Immediate Trigger.vi"("Instrument Handle In"=w441, "Error In"=w440) -> ("Instrument Handle Out"=w439:refnum<k21>, "Error Out"=w438:errorcluster)  [unwired: 12 in]
        n120 = call <vilib>:"MSO Run.vi"("Instrument Handle In"=w439, "Error In"=w438) -> ("Instrument Handle Out"=w436:refnum<k21>, "Error Out"=w437:errorcluster)  [unwired: 12 in]
        n121 = call <vilib>:"MSO Read.vi"("Instrument Handle In"=w436, "Error In"=w437) -> ("Instrument Handle Out"=w435:refnum<k21>, "Analog Waveforms"=→"波形图":waveform(dbl)[], "Error Out"=w434:errorcluster)  [unwired: 8 in, 3 out]
        n122 = call <vilib>:"MSO Stop.vi"("Instrument Handle In"=w435, "Error In"=w434) -> ("Instrument Handle Out"=w430:refnum<k21>, "Error Out"=w423:errorcluster)  [unwired: 12 in]
        n123 = call <vilib>:"FGEN Stop.vi"("Instrument Handle In"=w433, "Error In"=w423) -> ("Instrument Handle Out"=w432:refnum<k21>, "Error Out"=w412:errorcluster)  [unwired: 12 in]
        n124 = call <vilib>:"FGEN Close.vi"("Instrument Handle In"=w432, "Error In"=w412) -> ("Error Out"=w431:errorcluster)  [unwired: 13 in]
        n125 = call <vilib>:"MSO Close.vi"("Instrument Handle In"=w430, "Error In"=w431) -> ("Error Out"=w411:errorcluster)  [unwired: 13 in]
      }
    }
    n126 = Or(x=w51, y=w54) -> (x .or. y?=w53:bool)
    n127 = local write "测试进度"(w55) -> ()
  }
  n128 = call <vilib>:"DWF Dig Reset Instrument.vi"("Instrument Handle In"=w2, "Error In"=w5) -> ("Instrument Handle Out"=w1:u32, "Error Out"=w4:errorcluster)  [unwired: 12 in]
  n129 = call <vilib>:"DWF Dig Close.vi"("Instrument Handle In"=w1, "Error In"=w4) -> ("Error Out"=w3:errorcluster)  [unwired: 13 in]
  n130 = call <vilib>:"Dig Reset Instrument.vi"("Instrument Handle In"=w15, "Error In"=w3) -> ("Instrument Handle Out"=w25:refnum<k21>, "Error Out"=w24:errorcluster)  [unwired: 12 in]
  n131 = call <vilib>:"Dig Close.vi"("Instrument Handle In"=w25, "Error In"=w24) -> ("Error Out"=w22:errorcluster)  [unwired: 13 in]
  n132 = call <vilib>:"PS Reset Instrument.vi"("Instrument Handle In"=w23, "Error In"=w22) -> ("Instrument Handle Out"=w20:refnum<k21>, "Error Out"=w21:errorcluster)  [unwired: 12 in]
  n133 = call <vilib>:"PS Close.vi"("Instrument Handle In"=w20, "Error In"=w21) -> ("Error Out"=w19:errorcluster)  [unwired: 13 in]
  n134 = call <vilib>:"DMM Reset Instrument.vi"("Instrument Handle In"=w17, "Error In"=w19) -> ("Instrument Handle Out"=w16:refnum<k21>, "Error Out"=w18:errorcluster)  [unwired: 12 in]
  n135 = call <vilib>:"DMM Close.vi"("Instrument Handle In"=w16, "Error In"=w18) -> ("Error Out"=w26:errorcluster)  [unwired: 13 in]
  n136 = case shown="无错误" w26 {
    selector: w26 -> [_ w454]
    frame No Error {
      n137 = local write "测试进度"(u8 100 ("测试进度")) -> ()
    }
    frame Error {
      w455 = T6 3 items=["no dialog", "OK message", "continue or stop message", "OK message + warnings", "continue/stop + warnings"] ("type of dialog (OK msg:1)")
      n138 = call <vilib>:"Simple Error Handler.vi"("type of dialog (OK msg:1)"=w455, "error in (no error)"=w454) -> ()  [unwired: 3 in, 5 out]
    }
  }
